vi "ADC_Conversion y leer.vi"(0 "ftHandle_in 2":u32, 1 "Espera acceso USB":u32=10, 5 "Registro Conversion (0xD000)":u16=53248 format="%04x", 11 "error in 2":errorcluster) -> (4 "ftHandle_out":u32, 6 "Datos Canal (V)":dbl[](array[numeric]), 8 "Datos Canal":u16[](array[numeric]) format="%04x", 10 "Posible error":bool, 14 "Dout (sin tratar)":u8[](array[numeric])=[1, 0, 0, 0, 184, 0, 16, 224, 0, 2, 113, 76, 75, 64, 0, 0, 39, 0, 24, 52, 33, 241, 29, 50, 41, 102, 53, 71, 78, 101, 89, 183, 105, 43, 121, 27, 136, 207, 144, 0, 160, 0, 176, 0] format="%.0x", 15 "error out":errorcluster)   [LabVIEW 2019]
uses:
  Global cuenta erroes.vi
panel:
  out "lpBuffer_out":u8[](array[numeric])
  in  "Espera digitalización":u32
  in  "error in":errorcluster
  out "error out":errorcluster
  out "ftHandle_out":u32
  in  "ftHandle_in":u32
  in  "Registro Conversion":u8 format="%x"
  in  "Espera acceso USB:":u32
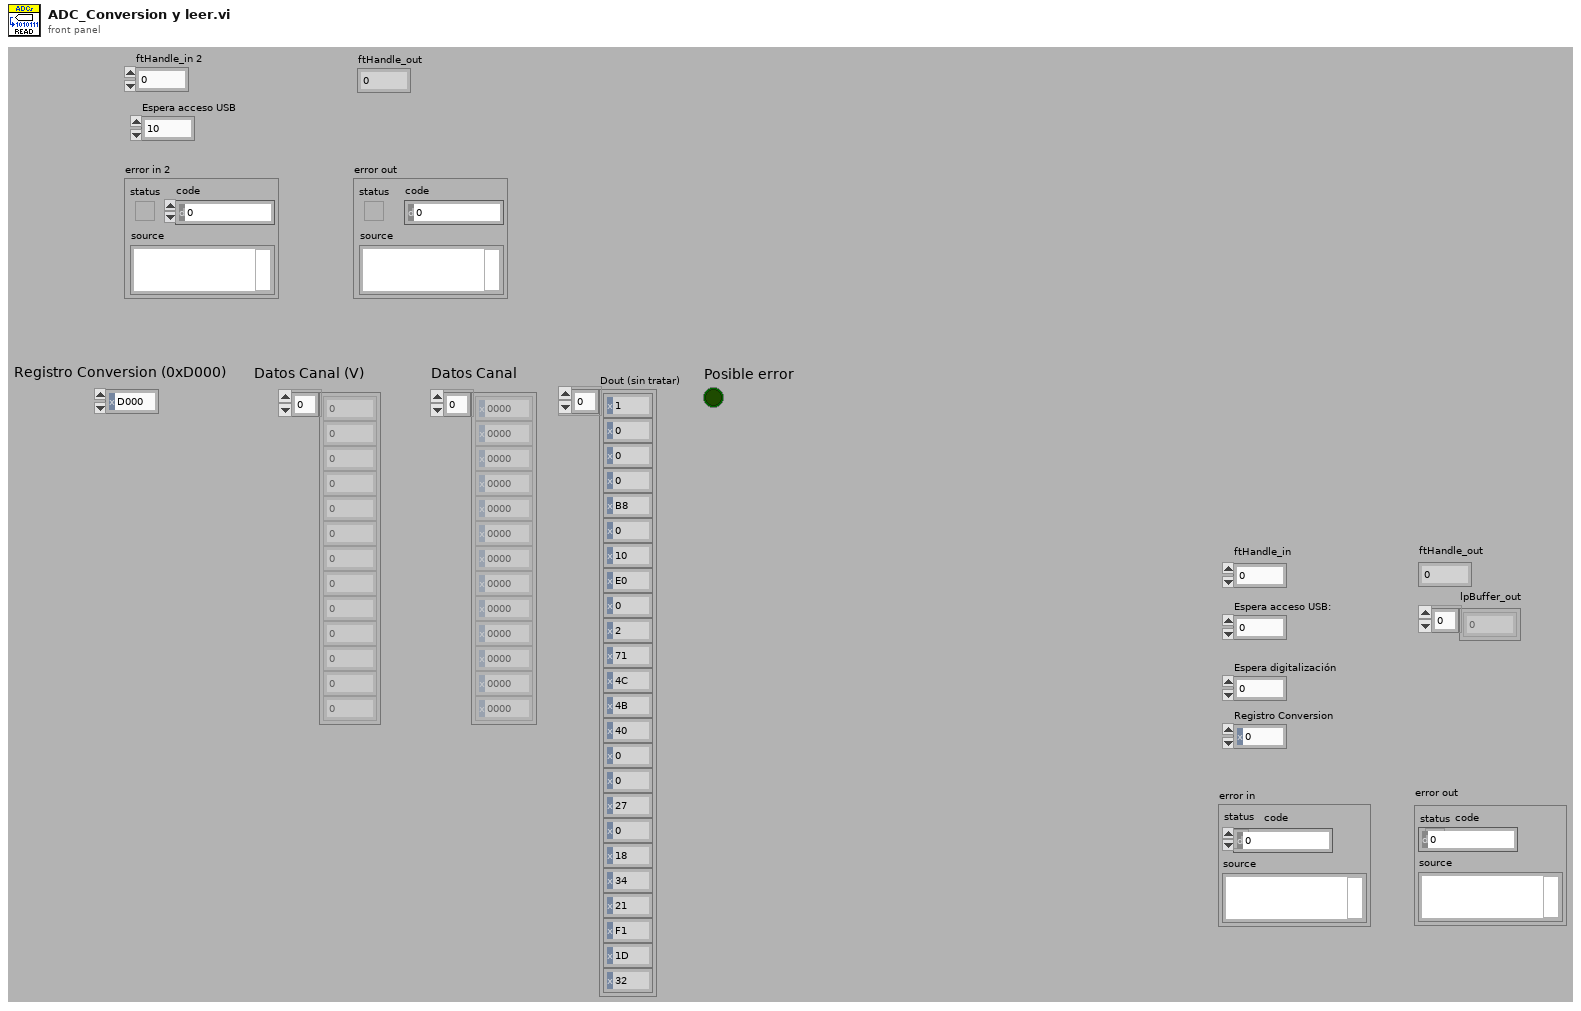
[diagram p1: front panel]
types:
  T1 = typedef "global erroes cluster.ctl" = cluster{"Errores FPGA":i32, "Errores Asic":i32, "Errores ADC adq":i32, "Errores ADC Asic":i32}
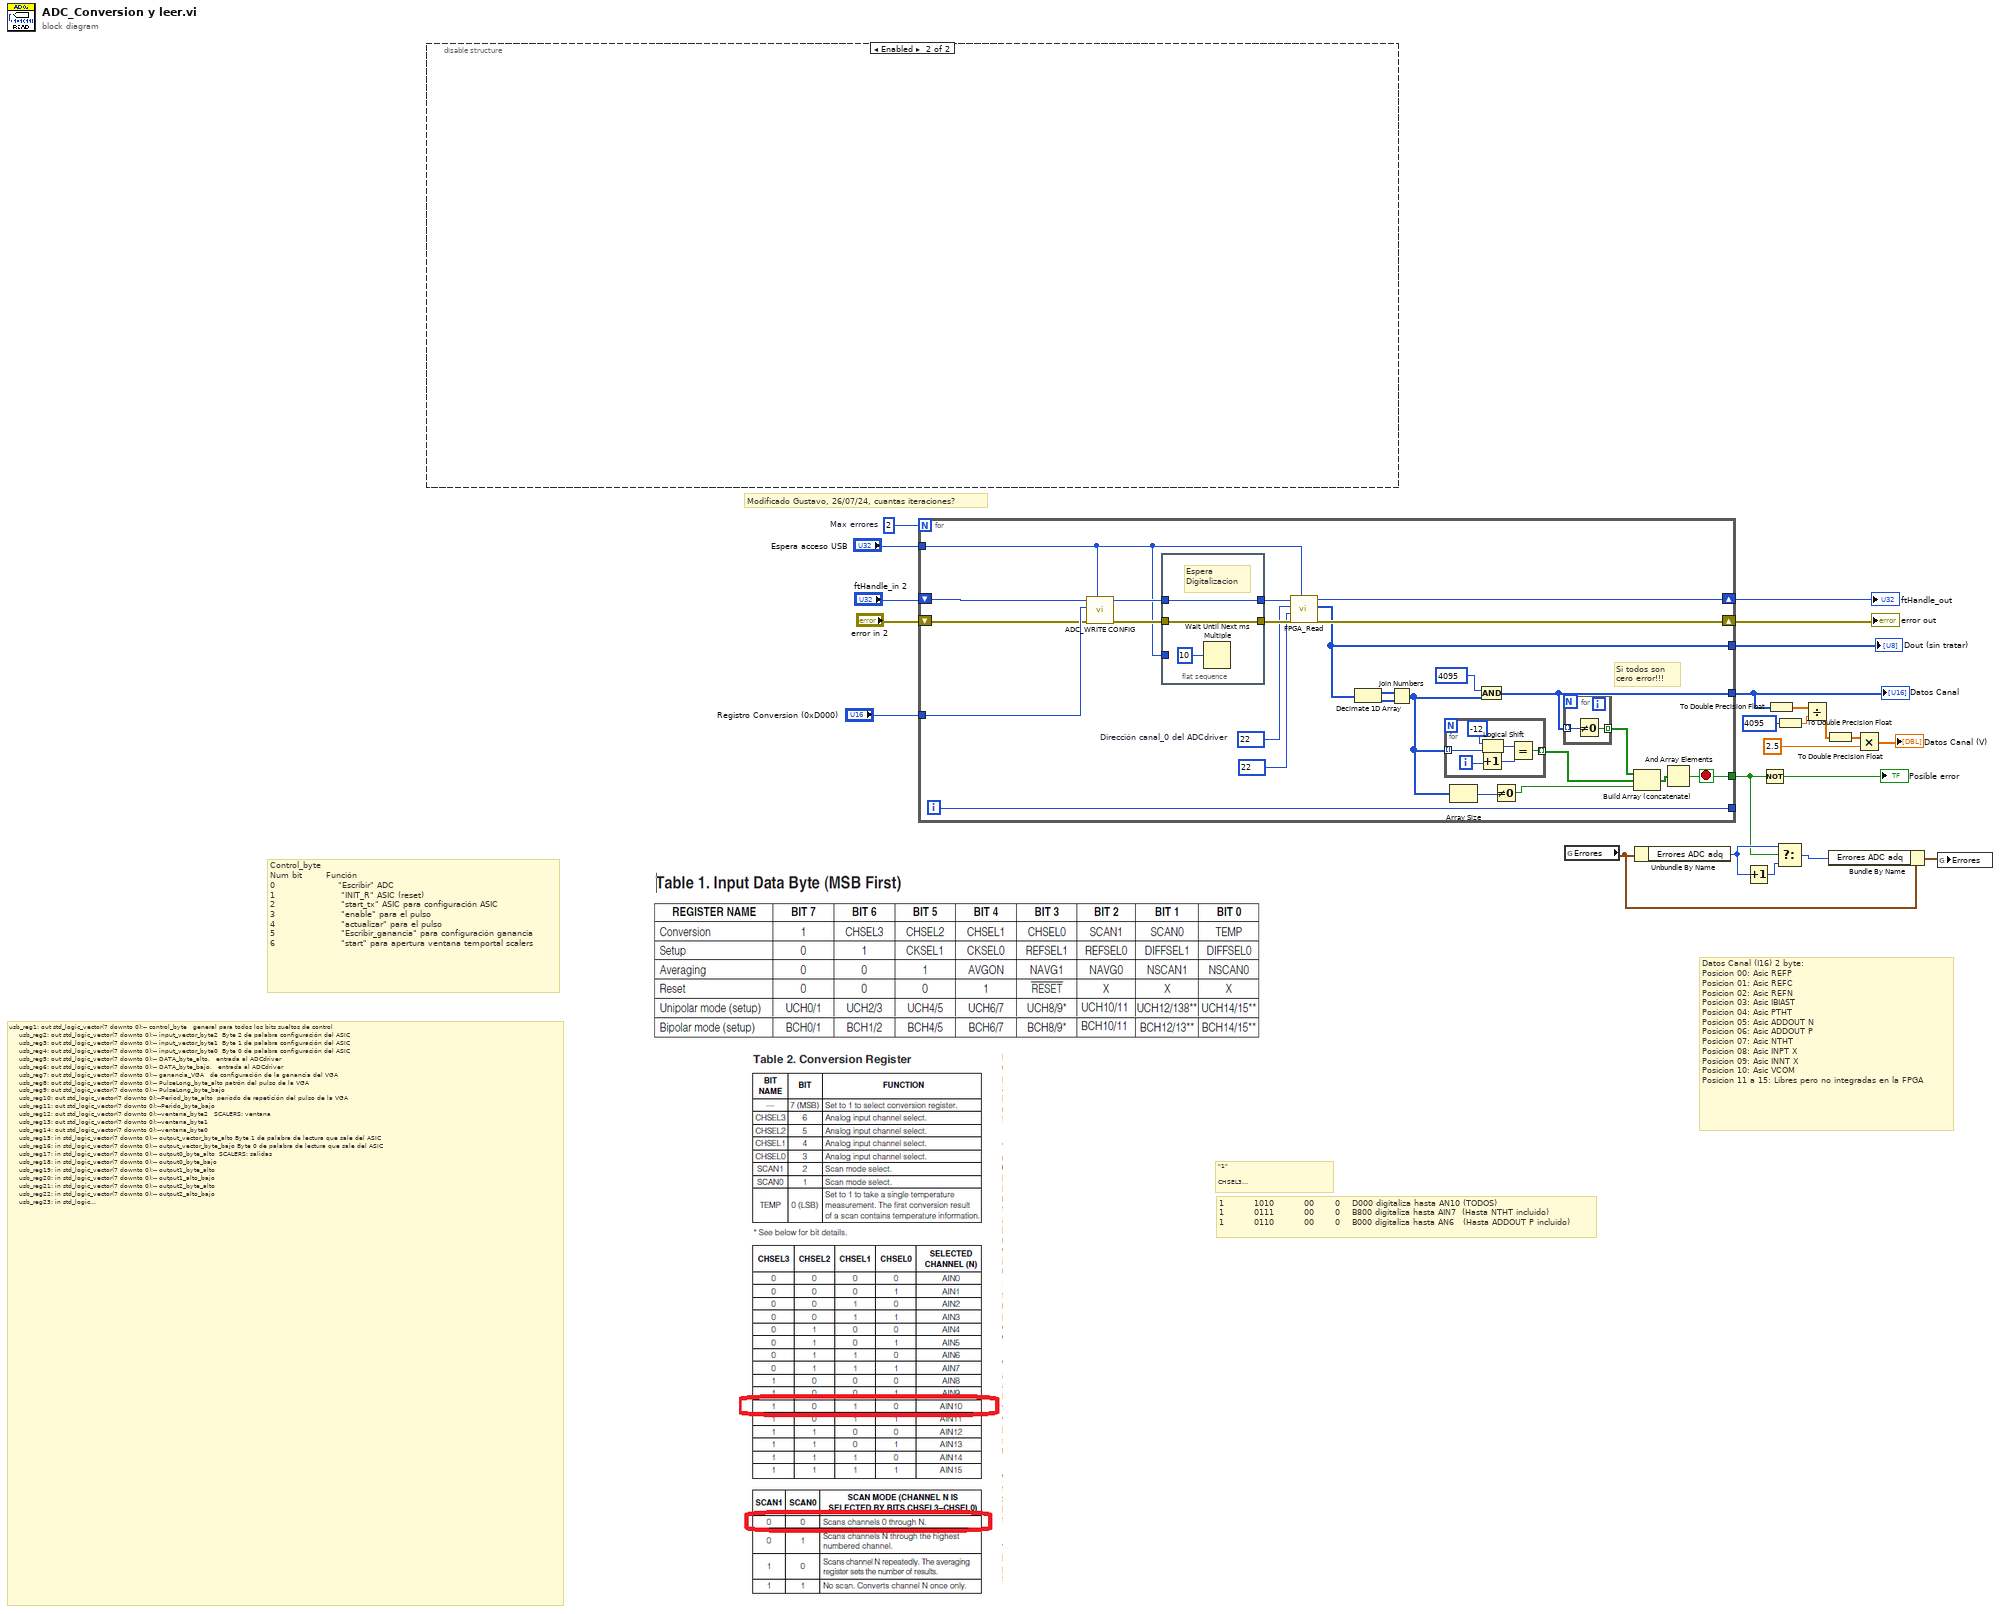
[diagram p0: block diagram]
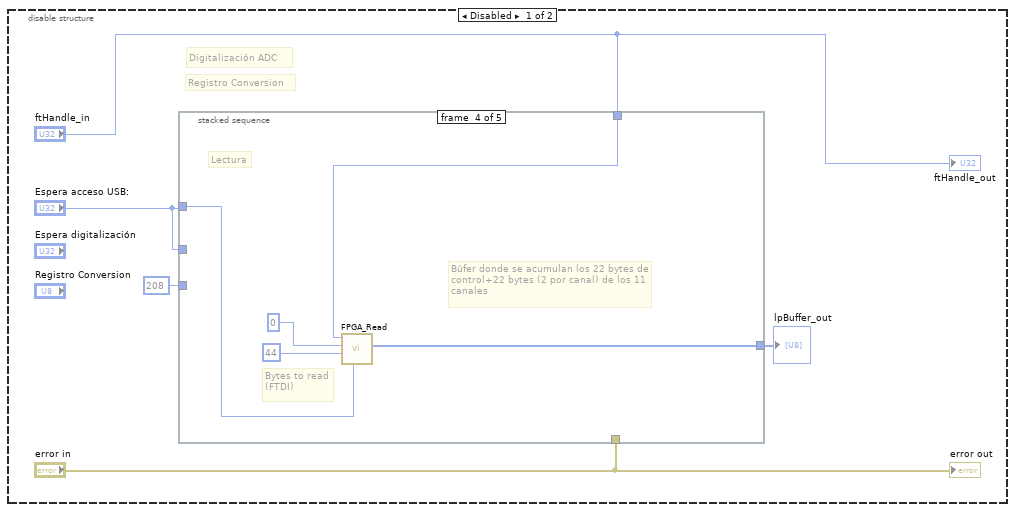
[diagram p2: hidden frame]
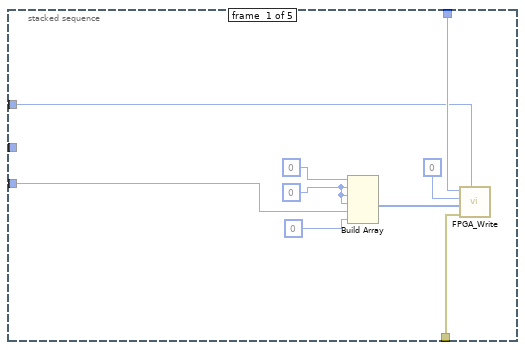
[diagram p3: hidden frame]
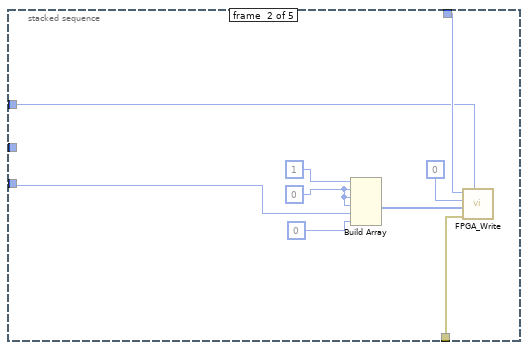
[diagram p4: hidden frame]
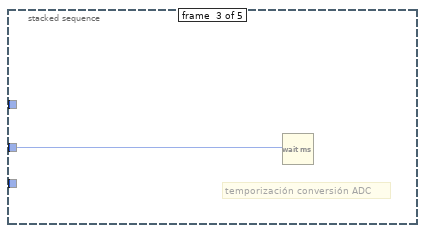
[diagram p5: hidden frame]
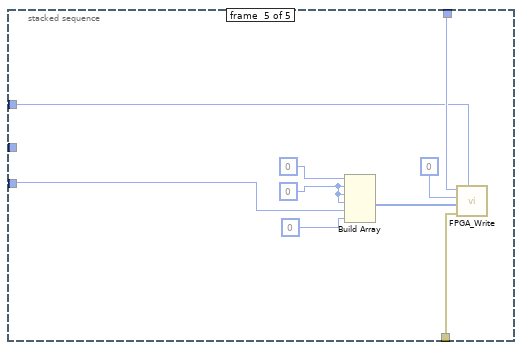
[diagram p6: hidden frame]
diagram:
  w16 = 2  # Max errores
  # "Modificado Gustavo, 26/07/24, cuantas iteraciones?"
  # "\"1\"\n\nCHSEL3\nCHSEL2\nCHSEL1\nCHSEL0\n\nSCAN1\nSCAN0\n\nTEMP"
  # "Datos Canal (I16) 2 byte:\nPosicion 00: Asic REFP\nPosicion 01: Asic REFC\nPosicion 02: Asic REFN\nPosicion 03: Asic IBIAST\nPosicion 04: Asic PTHT\nPosicion 05: Asic ADDOUT N\nPosicion 06: Asic ADDOUT P\nPosicion 07: Asic NTHT\nPosicion 08: Asic INPT X\nPosicion 09: Asic INNT X\nPosicion 10: Asic VCOM\nPosicion 11 a 15: Libres pero no integradas en la FPGA"
  # "1          1010          00       0    D000 digitaliza hasta AN10 (TODOS) \n1          0111          00       0    B800 digitaliza hasta AIN7  (Hasta NTHT incluido)\n1          0110          00       0    B000 digitaliza hasta AN6   (Hasta ADDOUT P incluido)"
  # "Control_byte\nNum bit        Función\n0                     \"Escribir\" ADC\n1                      \"INIT_R\" ASIC (reset)\n2                      \"start_tx\" ASIC para configuración ASIC\n3                      \"enable\" para el pulso\n4                      \"actualizar\" para el pulso\n5                      \"Escribir_ganancia\" para configuración ganancia\n6                      \"start\" para apertura ventana temportal scalers"
  # "usb_reg1: out std_logic_vector(7 downto 0);-- control_byte\t\t\tgeneral para todos los bits sueltos de control\n\t\t\t  usb_reg2: out std_logic_vector(7 downto 0);-- input_vector_byte2 \tByte 2 de palabra configuración del ASIC\n\t\t\t  usb_reg3: out std_logic_vector(7 downto 0);-- input_vector_byte1 \tByte 1 de palabra configuración del ASIC\n\t\t\t  usb_reg4: out std_logic_vector(7 downto 0);-- input_vector_byte0 \tByte 0 de palabra configuración del ASIC\n\t\t\t  usb_reg5: out std_logic_vector(7 downto 0);-- DATA_byte_alto, \t\tentrada al ADCdriver\n\t\t\t  usb_reg6: out std_logic_vector(7 downto 0);-- DATA_byte_bajo, \t\tentrada al ADCdriver\n\t\t\t  usb_reg7: out std_logic_vector(7 downto 0);-- ganancia_VGA\t\t\tde configuración de la ganancia del VGA\n\t\t\t  usb_reg8: out std_logic_vector(7 downto 0);-- PulseLong_byte_alto\tpatrón del pulso de la VGA\n\t\t\t  usb_reg9: out std_logic_vector(7 downto 0);-- PulseLong_byte_bajo\n\t\t\t  usb_reg10: out std_logic_vector(7 downto 0);--Period_byte_alto\t\tperíodo de repetición del pulso de la VGA\n\t\t\t  usb_reg11: out std_logic_vector(7 downto 0);--Perido_byte_bajo\n\t\t\t  usb_reg12: out std_logic_vector(7 downto 0);--ventana_byte2\t\t\tSCALERS: ventana\n\t\t\t  usb_reg13: out std_logic_vector(7 downto 0);--ventana_byte1\t\n\t\t\t  usb_reg14: out std_logic_vector(7 downto 0);--ventana_byte0\n\t\t\t  usb_reg15: in std_logic_vector(7 downto 0);-- output_vector_byte_alto\tByte 1 de palabra de lectura que sale del ASIC\n\t\t\t  usb_reg16: in std_logic_vector(7 downto 0);-- output_vector_byte_bajo\tByte 0 de palabra de lectura que sale del ASIC\n\t\t\t  usb_reg17: in std_logic_vector(7 downto 0);-- output0_byte_alto\t\tSCALERS: salidas\n\t\t\t  usb_reg18: in std_logic_vector(7 downto 0);-- output0_byte_bajo\n\t\t\t  usb_reg19: in std_logic_vector(7 downto 0);-- output1_byte_alto\n\t\t\t  usb_reg20: in std_logic_vector(7 downto 0);-- output1_alto_bajo \n\t\t\t  usb_reg21: in std_logic_vector(7 downto 0);-- output2_byte_alto \n\t\t\t  usb_reg22: in std_logic_vector(7 downto 0);-- output2_alto_bajo \n\t\t\t  usb_reg23: in std_logic_vector(7 downto 0);-- para el canal_0 del ADCdriver\n\t\t\t  usb_reg24: in std_logic_vector(7 downto 0);\n\t\t\t  usb_reg25: in std_logic_vector(7 downto 0);-- para el canal_1 del ADCdriver\n\t\t\t  usb_reg26: in std_logic_vector(7 downto 0);\n\t\t\t  usb_reg27: in std_logic_vector(7 downto 0);-- para el canal_2 del ADCdriver\n\t\t\t  usb_reg28: in std_logic_vector(7 downto 0);\n\t\t\t  usb_reg29: in std_logic_vector(7 downto 0);-- para el canal_3 del ADCdriver\n\t\t\t  usb_reg30: in std_logic_vector(7 downto 0);\n\t\t\t  usb_reg31: in std_logic_vector(7 downto 0);-- para el canal_4 del ADCdriver\n\t\t\t  usb_reg32: in std_logic_vector(7 downto 0);\n\t\t\t  usb_reg33: in std_logic_vector(7 downto 0);-- para el canal_5 del ADCdriver\n\t\t\t  usb_reg34: in std_logic_vector(7 downto 0);\n\t\t\t  usb_reg35: in std_logic_vector(7 downto 0);-- para el canal_6 del ADCdriver\n\t\t\t  usb_reg36: in std_logic_vector(7 downto 0);\n\t\t\t  usb_reg37: in std_logic_vector(7 downto 0);-- para el canal_7 del ADCdriver\n\t\t\t  usb_reg38: in std_logic_vector(7 downto 0);\n\t\t\t  usb_reg39: in std_logic_vector(7 downto 0);-- para el canal_8 del ADCdriver\n\t\t\t  usb_reg40: in std_logic_vector(7 downto 0);\n\t\t\t  usb_reg41: in std_logic_vector(7 downto 0);-- para el canal_9 del ADCdriver\n\t\t\t  usb_reg42: in std_logic_vector(7 downto 0);\n\t\t\t  usb_reg43: in std_logic_vector(7 downto 0);-- para el canal_10 del ADCdriver\n\t\t\t  usb_reg44: in std_logic_vector(7 downto 0)--;"
  n1 = disable-structure shown="Enabled" {
    frame Disabled {
      # "Registro Conversion"
      # "Digitalización ADC"
      n2 = stacked-sequence {
        tunnel: "ftHandle_in" -> [w34 w41 _ w52 w55]
        tunnel: "Espera acceso USB:" -> [w29 w38 _ w48 w53]
        tunnel: u8 208 ("Registro Conversion") -> [w31 w40 _ _ w56]
        tunnel: "error in" -> [w30 w39 _ _ w54]
        tunnel: "Espera acceso USB:" -> [_ _ w47 _ _]
        tunnel: [_ _ _ w51 _] -> w26
        frame #0 {
          w33 = u8 0 ("x")
          n3 = Build Array(u8 0 ("x"), w33, w33, w33, w31, u8 0 ("x")) -> (w36:u8[])
          n4 = call "FPGA_Write.vi"("Espera acceso USB"=w29, "error in"=w30, "Bytes de escritura"=w36, "Dirección base"=u8 0 ("x"), "ftHandle_in"=w34) -> ()  [unwired: 1 in, 4 out]
        }
        frame #1 {
          w43 = u8 0 ("x")
          n5 = Build Array(u8 1 ("x"), w43, w43, w43, w40, u8 0 ("x")) -> (w45:u8[])
          n6 = call "FPGA_Write.vi"("Espera acceso USB"=w38, "error in"=w39, "Bytes de escritura"=w45, "Dirección base"=u8 0 ("x"), "ftHandle_in"=w41) -> ()  [unwired: 1 in, 4 out]
        }
        frame #2 {
          # "temporización conversión ADC"
          n7 = Wait (ms)(milliseconds to wait=w47) -> ()  [unwired: 1 out]
        }
        frame #3 {
          # "Búfer donde se acumulan los 22 bytes de control+22 bytes (2 por canal) de los 11 canales"
          # "Bytes to read (FTDI)"
          # "Lectura"
          n8 = call "FPGA_Read.vi"("Espera acceso USB"=w48, "Numero Bytes"=u16 44 ("devNum_in"), "Dirección base"=u16 0 ("devNum_in"), "ftHandle_in"=w52) -> ("lpBuffer_out"=w51:u8[])  [unwired: 3 in, 4 out]
        }
        frame #4 {
          w58 = u8 0 ("x")
          n9 = Build Array(u8 0 ("x"), w58, w58, w58, w56, u8 0 ("x")) -> (w60:u8[])
          n10 = call "FPGA_Write.vi"("Espera acceso USB"=w53, "error in"=w54, "Bytes de escritura"=w60, "Dirección base"=u8 0 ("x"), "ftHandle_in"=w55) -> ()  [unwired: 1 in, 4 out]
        }
      }
      "lpBuffer_out" <- w26
      "ftHandle_out" <- "ftHandle_in"
      "error out" <- "error in"
    }
    frame Enabled {
    }
  }
  n11 = for {
    N: w16 -> [_]
    tunnel: "Registro Conversion (0xD000)" -> [w86]
    tunnel: "Espera acceso USB" -> [w79]
    tunnel: [w74] -> w17
    tunnel: [w70] -> w12
    shift-right: [w81] -> w20
    shift-left: "ftHandle_in 2" -> [w73]
    shift-right: [w80] -> w19
    shift-left: "error in 2" -> [w72]
    tunnel: [w69] -> w1
    tunnel: [w71] -> _
    i -> [w71]
    stop <- w69 stop-if-true
    w78 = u8 22  # Dirección canal_0 del ADCdriver
    # "Si todos son cero error!!!"
    n12 = call "ADC_WRITE CONFIG.vi"("Espera acceso USB"=w79, "error in 2"=w72, "Dac Data IN"=w86, "ftHandle_in 2"=w73) -> ("error out"=w84:errorcluster, "ftHandle_out"=w85:u32)  [unwired: 6 in]
    n13 = flat-sequence {
      tunnel: [w97] -> w82
      tunnel: w85 -> [w97]
      tunnel: w84 -> [w96]
      tunnel: [w96] -> w83
      tunnel: w79 -> [_]
      frame #0 {
        # "Espera\nDigitalizacion"
        n14 = Wait Until Next ms Multiple(millisecond multiple=u32 10) -> ()  [unwired: 1 out]
      }
    }
    n15 = call "FPGA_Read.vi"("Espera acceso USB"=w79, "error in"=w83, "Numero Bytes"=u8 22 ("Dirección base"), "Dirección base"=w78, "ftHandle_in"=w82) -> ("error out"=w80:errorcluster, "lpBuffer_out"=w74:u8[], "ftHandle_out"=w81:u32)  [unwired: 2 in, 2 out]
    n16 = Decimate 1D Array(w74) -> (w76:u8[], w75:u8[])
    n17 = Join Numbers(hi=w76, lo=w75) -> ((hi.lo)=w64:u16[])
    n18 = for {
      tunnel: w64 -> [w89] mode=indexing
      tunnel: [w90] -> w67 mode=indexing
      i -> [w92]
      n19 = Increment(x=w92) -> (x+1=w91:i32)
      n20 = Logical Shift(y=i8 -12, x=w89) -> (x << y=w87:u16)
      n21 = Equal?(x=w87, y=w91) -> (x = y?=w90:bool)
    }
    n22 = Array Size(array=w64) -> (size(s)=w63:i32)
    n23 = And(x=u16 4095, y=w64) -> (x .and. y?=w70:u16[])
    n24 = Not Equal To 0?(x=w63) -> (x != 0?=w62:bool)
    n25 = for {
      tunnel: w70 -> [w94] mode=indexing
      tunnel: [w93] -> w65 mode=indexing
      n26 = Not Equal To 0?(x=w94) -> (x != 0?=w93:bool)
    }
    n27 = Build Array (concatenate)(w65, w67, w62) -> (w66:bool[])
    n28 = And Array Elements(Boolean array=w66) -> (logical AND=w69:bool)
  }
  "error out" <- w19
  "ftHandle_out" <- w20
  "Dout (sin tratar)" <- w17
  "Datos Canal" <- w12
  n29 = global read "Global cuenta erroes.vi" "Errores"() -> (w7:T1)
  n30 = Unbundle By Name(w7) -> ("Errores ADC adq"=w3:i32)
  n31 = Increment(x=w3) -> (x+1=w4:i32)
  n32 = Not(x=w1) -> (.not. x?=→"Posible error":bool)
  n33 = To Double Precision Float(number=w12) -> (double precision float=w10:dbl[])
  n34 = Select(t=w3, s=w1, f=w4) -> (s? t:f=w2:i32)
  n35 = To Double Precision Float(number=u16 4095 ("index")) -> (double precision float=w9:dbl)
  n36 = Divide(x=w10, y=w9) -> (x/y=w14:dbl[])
  n37 = To Double Precision Float(number=w14) -> (double precision float=w11:dbl[])
  n38 = Bundle By Name(cluster=w7, "Errores ADC adq"=w2) -> (w6:T1)
  n39 = Multiply(x=w11, y=2.5 ("index")) -> (x*y=→"Datos Canal (V)":dbl[])
  n40 = global write "Global cuenta erroes.vi" "Errores"(w6) -> ()
